vi "GetMetricTdmsProps.vi"(11 "metric":T1) -> (1 "TdmsUnitValue":string, 2 "TdmsDisplayName":string, 3 "TdmsPropName":string)   [LabVIEW 2017, in "EmsaAnalysis.lvlib"]
uses:
  <vilib>/addons/InsightCM/Devices/Shared/Emsa/EmsaAnalysis/EmsaAnalysis.lvlib
  <vilib>/addons/InsightCM/MessageBus/Base/controls/KeyValuePair.ctl
  <vilib>/addons/InsightCM/MessageBus/Base/controls/MetricDefinitionInstance.ctl
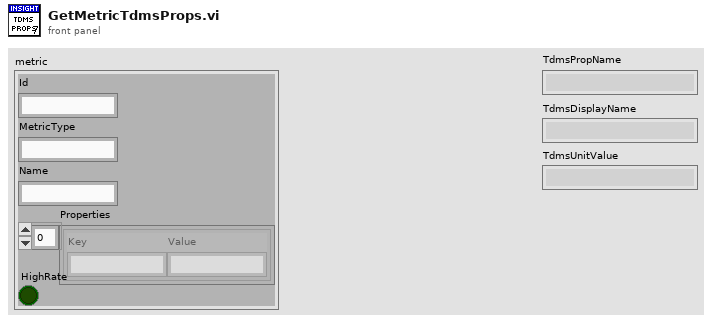
[diagram p1: front panel]
types:
  T1 = typedef "MetricDefinitionInstance.ctl" = cluster{"Id":string, "MetricType":string, "Name":string, "Properties":T2[], "HighRate":bool}
  T2 = typedef "KeyValuePair.ctl" = cluster{"Key":string, "Value":string}
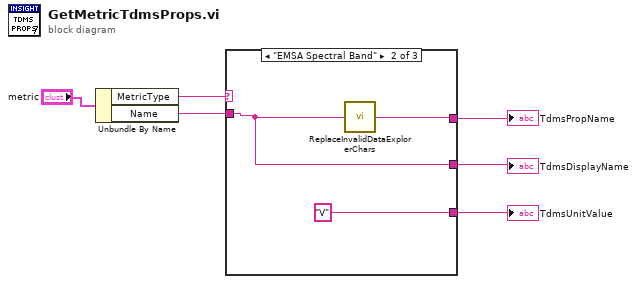
[diagram p0: block diagram]
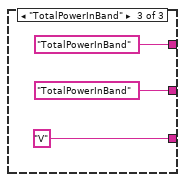
[diagram p3: hidden frame]
diagram:
  n1 = Unbundle By Name("metric") -> ("MetricType"=w5:string, "Name"=w1:string)
  n2 = case shown="\"EMSA Spectral Band\"" w5 {
    tunnel: [_ w8 "TotalPowerInBand"] -> w4
    tunnel: [_ w7 "TotalPowerInBand"] -> w3
    tunnel: [_ "V" "V"] -> w2
    tunnel: w1 -> [_ w7 _]
    frame "", Default {
    }
    frame "EMSA Spectral Band" {
      n3 = call <vilib>:"ReplaceInvalidDataExplorerChars.vi"("input string"=w7) -> ("result string"=w8:string)  [unwired: 4 in]
    }
    frame "TotalPowerInBand" {
    }
  }
  "TdmsPropName" <- w4
  "TdmsDisplayName" <- w3
  "TdmsUnitValue" <- w2
